vi "Init Rx UDP Connection.vi"(8 "error in (no error)":errorcluster, 11 "Rx Loop Data in":T1) -> (0 "error out":errorcluster, 3 "Rx Loop Data out":T1)   [LabVIEW 2015, in "UDP-Custom-Device Engine.lvlib"]
uses:
  UDP-Custom-Device Engine.lvlib
  Rx Loop Data.ctl
  <vilib>/NI/NIVS Inline Async API/_Data Access Engine/Data Access Engine/Types/Write.DVR.ctl
  <vilib>/NI/NIVS Inline Async API/_Data Access Engine/Access Type Classes/Write/Write.lvclass
  <vilib>/NI/NIVS Inline Async API/_Data Access Engine/Data Access Engine/Data Access Engine.lvclass
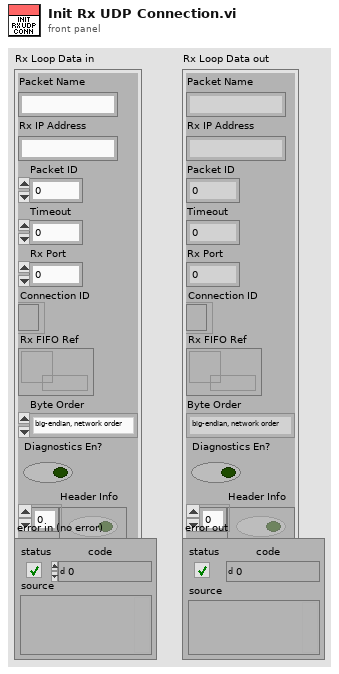
[diagram p1: front panel]
types:
  T1 = typedef "UDP-Custom-Device Engine.lvlib/Rx Loop Data.ctl" = cluster{"Packet Name":string, "Rx IP Address":string, "Packet ID":i32, "Timeout":i32, "Rx Port":i32, "Connection ID":refnum<k16>, "Rx FIFO Ref":T2, "Byte Order":enum16{"big-endian, network order", "native, host order", "little-endian"}, "Diagnostics En?":bool, "Header Info":bool[]}
  T2 = typedef "Data Access Engine.lvlib/Data Access Engine.lvclass/Write.DVR.ctl" = refnum<data-value>
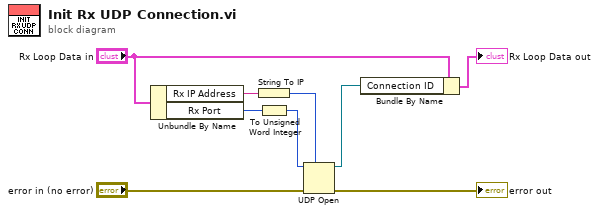
[diagram p0: block diagram]
diagram:
  n1 = Unbundle By Name("Rx Loop Data in") -> ("Rx IP Address"=w5:string, "Rx Port"=w6:i32)
  n2 = String To IP(1:w5) -> (0:w4:u32)
  n3 = To Unsigned Word Integer(number=w6) -> (unsigned 16bit integer=w1:u16)
  n4 = UDP Open(7:w4, 8:"error in (no error)", 11:w1) -> (port=w3:refnum<k16>, 0:→"error out":errorcluster)  [unwired: 2 in, 1 out]
  n5 = Bundle By Name(cluster="Rx Loop Data in", "Connection ID"=w3) -> (→"Rx Loop Data out":T1)
